vi "GetControlRefFromControlArray.vi"(0 "Controls[]":refnum<vi>[](array[refnum]), 7 "Control Name":string, 11 "error In":errorcluster) -> (4 "Remaining Controls[]":refnum<vi>[](array[refnum]), 8 "Target Control":refnum<vi>, 15 "error out":errorcluster)   [LabVIEW 2016]
doc: "This VI gives the desired control reference from the array of control references"
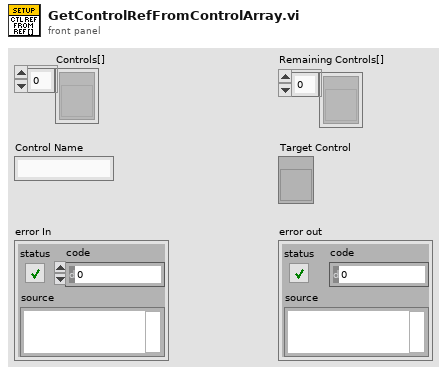
[diagram p1: front panel]
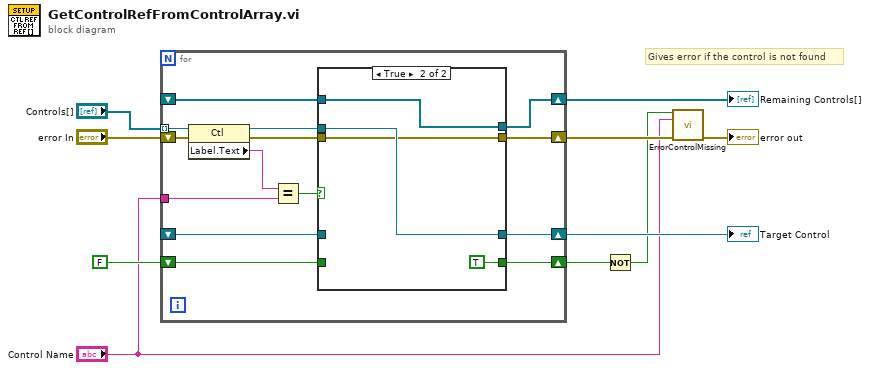
[diagram p0: block diagram]
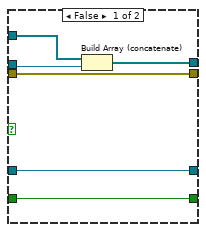
[diagram p2: hidden frame]
diagram:
  # "Gives error if the control is not found"
  n1 = for {
    tunnel: "Controls[]" -> [w24] mode=indexing
    tunnel: "Control Name" -> [w22]
    shift-right: [w19] -> w9
    shift-left: _ -> [w18]
    shift-right: [w17] -> w8
    shift-left: _ -> [w16]
    shift-right: [w14] -> w3
    shift-left: FALSE -> [w15]
    shift-right: [w11] -> w5
    shift-left: "error In" -> [w13]
    n2 = property class="Ctl"(reference=w24, error in=w13) -> (reference out=w20:refnum<vi>, error out=w12:errorcluster, "Label.Text"=w23:string)
    n3 = Equal?(x=w23, y=w22) -> (x = y?=w21:bool)
    n4 = case shown="True" w21 {
      tunnel: w20 -> [w29 w33]
      tunnel: [w25 w34] -> w19
      tunnel: w18 -> [w30 w34]
      tunnel: [w28 w33] -> w17
      tunnel: w16 -> [w28 _]
      tunnel: w15 -> [w27 _]
      tunnel: [w27 TRUE] -> w14
      tunnel: w12 -> [w26 w31]
      tunnel: [w26 w31] -> w11
      frame False {
        n5 = Build Array (concatenate)(w30, w29) -> (w25:refnum<vi>[])
      }
      frame True {
      }
    }
  }
  "Remaining Controls[]" <- w9
  "Target Control" <- w8
  n6 = Not(x=w3) -> (.not. x?=w1:bool)
  n7 = call "ErrorControlMissing.vi"("Create Error?"=w1, "Control Name"="Control Name", "error in"=w5) -> ("error out"=→"error out":errorcluster)  [unwired: 12 in]
